vi "Installed Distributions OLD.vi"() -> ()   [LabVIEW 2015]
uses:
  <vilib>/registry/registry.llb/Registry SAM.ctl
  <vilib>/registry/registry.llb/Read Registry Value Simple STR.vi
panel:
  in  "Registry Key":string="SOFTWARE\\National Instruments\\Common\\Installer\\Distributions"
  out "Paths To Installers":string
  out "Dist Names":string[](array[string])
  out "Dist Paths":string[](array[string])
  out "error out":errorcluster
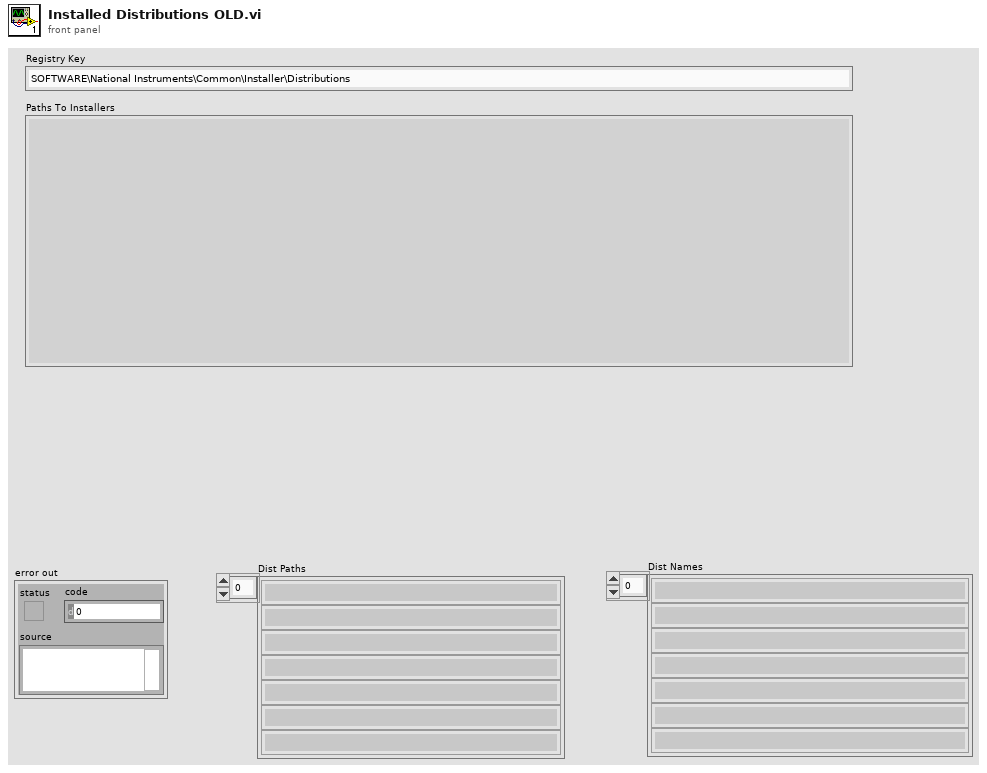
[diagram p1: front panel]
types:
  T1 = typedef "Registry SAM.ctl" = enum32{"KEY_QUERY_VALUE", "KEY_SET_VALUE", "KEY_CREATE_SUB_KEY", "KEY_ENUMERATE_SUB_KEYS", "KEY_NOTIFY", "KEY_CREATE_LINK", "KEY_READ", "KEY_WRITE", "KEY_ALL_ACCESS", "KEY_READ | KEY_WRITE"}
  T2 = typedef "Registry refnum.ctl" = refnum<k1>
  T3 = cluster{"numSubKeys":i32, "maxSubKeyLen":i32, "maxSubKeyClassLen":i32}
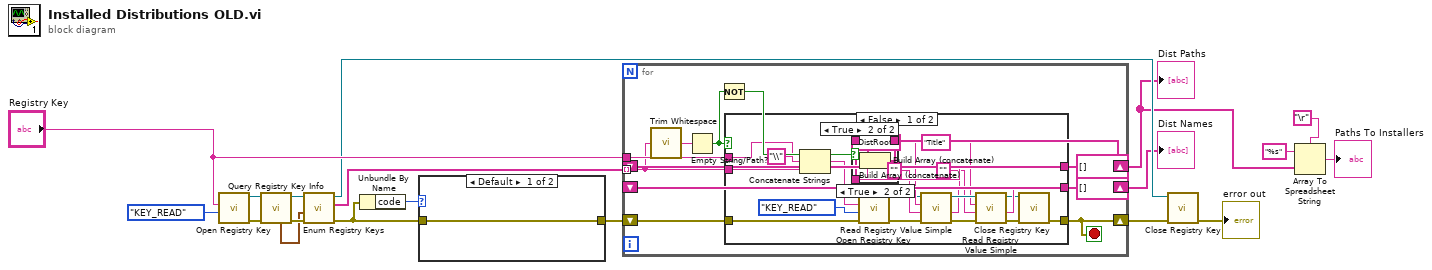
[diagram p0: block diagram]
diagram:
  n1 = call <vilib>:"Open Registry Key.vi"("security access mask (KEY_READ | KEY_WRITE)"=Registry_SAM."KEY_READ", "subkey"="Registry Key") -> ("error out"=w9:errorcluster, "refnum out"=w11:T2)  [unwired: 8 in]
  n2 = call <vilib>:"Query Registry Key Info.vi"("error in (no error)"=w9, "refnum"=w11) -> ("error out"=w8:errorcluster, "refnum out"=w10:T2, "subkey info"=w7:T3)  [unwired: 5 in, 2 out]
  n3 = call <vilib>:"Enum Registry Keys.vi"("error in (no error)"=w8, "subkey info"=w7, "refnum"=w10) -> ("error out"=w12:errorcluster, "subkeys"=w20:string[], "refnum out"=w16:T2)  [unwired: 6 in]
  n4 = Unbundle By Name(w12) -> ("code"=w14:i32)
  n5 = case shown="Default" w14 {
    tunnel: [w22 _] -> w13
    tunnel: w12 -> [w22 _]
    frame Default {
    }
    frame -605 {
      # "This case is when you have \nless than 100 distirbutions\ninstalled"
    }
  }
  n6 = for {
    tunnel: w20 -> [w30] mode=indexing
    tunnel: "Registry Key" -> [w35]
    shift-right: [w31] -> w18
    shift-left: w13 -> [w34]
    shift-right: [w25] -> w5
    shift-left: string[] [] ("Array") -> [w26]
    shift-right: [w23] -> w15
    shift-left: string[] [] ("Array") -> [w24]
    stop <- w31 stop-if-true
    n7 = call <vilib>:"Trim Whitespace.vi"("string"=w30) -> ("trimmed string"=w29:string)  [unwired: 1 in]
    n8 = Empty String/Path?(string/path=w29) -> (empty?=w28:bool)
    n9 = Not(x=w28) -> (.not. x?=w27:bool)
    n10 = case shown="False" w28 {
      tunnel: w35 -> [w61 _]
      tunnel: w30 -> [w60 _]
      tunnel: w34 -> [w57 _]
      tunnel: [w49 _] -> w33
      tunnel: [w45 _] -> w31
      tunnel: [w47 _] -> w32
      frame False {
        n11 = Concatenate Strings(w61, "\\" ("string"), w60) -> (w59:string)
        n12 = call <vilib>:"Open Registry Key.vi"("error in (no error)"=w57, "security access mask (KEY_READ | KEY_WRITE)"=Registry_SAM."KEY_READ", "subkey"=w59) -> ("error out"=w56:errorcluster, "refnum out"=w53:T2)  [unwired: 7 in]
        n13 = call-poly <vilib>:"Read Registry Value Simple.vi"("error in (no error)"=w56, "default data"="", "value"="DistRoot", "refnum"=w53) -> ("error out"=w48:errorcluster, "String/Binary data"=w49:string, "refnum out"=w52:T2)  [unwired: 2 in, 1 out]
        n14 = call-poly <vilib>:"Read Registry Value Simple.vi"("error in (no error)"=w48, "default data"="", "value"="Title", "refnum"=w52) -> ("error out"=w46:errorcluster, "String/Binary data"=w47:string, "refnum out"=w44:T2)  [unwired: 2 in, 1 out]
        n15 = call <vilib>:"Close Registry Key.vi"("error in (no error)"=w46, "refnum"=w44) -> ("error out"=w45:errorcluster)  [unwired: 5 in]
      }
      frame True {
      }
    }
    n16 = case shown="True" w27 {
      tunnel: w24 -> [w36 w38]
      tunnel: w32 -> [_ w37]
      tunnel: [w36 w39] -> w23
      frame False {
      }
      frame True {
        n17 = Build Array (concatenate)(w38, w37) -> (w39:string[])
      }
    }
    n18 = case shown="True" w27 {
      tunnel: w26 -> [w40 w42]
      tunnel: w33 -> [_ w41]
      tunnel: [w40 w43] -> w25
      frame False {
      }
      frame True {
        n19 = Build Array (concatenate)(w42, w41) -> (w43:string[])
      }
    }
  }
  "Dist Paths" <- w5
  "Dist Names" <- w15
  n20 = call <vilib>:"Close Registry Key.vi"("error in (no error)"=w18, "refnum"=w16) -> ("error out"=→"error out":errorcluster)  [unwired: 5 in]
  n21 = Array To Spreadsheet String(delimiter (Tab)="\r", array=w5, 3:"%s" ("format string")) -> (spreadsheet string=→"Paths To Installers":string)
